vi "Count UP.vi"() -> (0 "Count Up":i32)   [LabVIEW 2014]
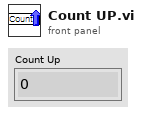
[diagram p1: front panel]
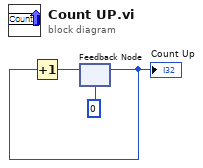
[diagram p0: block diagram]
diagram:
  n1 = feedback #1(0) -> (w2:i32)
  "Count Up" <- w2
  n2 = Increment(x=w2) -> (x+1=w1:i32)
  n3 = feedback-in #1(w1) -> ()
